vi "Receive.vi"(11 "jettl in":refnum<class "jettl.lvclass">) -> (2 "Msg":refnum<class "Msg Strategy.lvclass">, 3 "jettl out":refnum<class "jettl.lvclass">)   [LabVIEW 2021, in "jettl.lvlib" / "jettl.lvclass"]
uses:
  jettl.lvclass
  Msg Strategy/Msg Strategy.lvclass
  jettl.lvclass/jettl.ctl
  State/State/State.lvclass
  jettl.lvlib
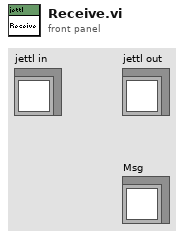
[diagram p1: front panel]
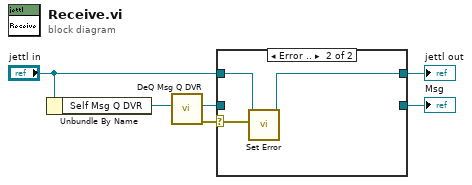
[diagram p0: block diagram]
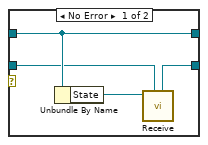
[diagram p2: hidden frame]
diagram:
  n1 = Unbundle By Name("jettl in") -> ("Self Msg Q DVR"=w6:refnum<data-value>)
  n2 = call "DeQ Msg Q DVR.vi"("Msg Q DVR"=w6) -> ("error out"=w5:errorcluster, "Msg"=w3:refnum<class "Msg Strategy.lvclass">)  [unwired: 9 in]
  n3 = case shown="Error .." w5 {
    selector: w5 -> [_ w11]
    tunnel: [w7 _] -> w4
    tunnel: w3 -> [w8 _]
    tunnel: "jettl in" -> [w9 w13]
    tunnel: [w9 w12] -> w1
    frame No Error {
      n4 = Unbundle By Name(w9) -> ("State"=w10:refnum<class "State.lvclass">)
      n5 = call-dynamic "Receive.vi"("Msg in"=w8, "State in"=w10) -> ("Msg out"=w7:refnum<class "Msg Strategy.lvclass">)  [unwired: 9 in]
    }
    frame Error {
      n6 = call-dynamic "Set Error.vi"("Error"=w11, "jettl in"=w13) -> ("jettl out"=w12:refnum<class "jettl.lvclass">)  [unwired: 9 in]
    }
  }
  "Msg" <- w4
  "jettl out" <- w1
